vi "Build RPC Request.vi"(10 "Command Params":string[][](array[string]), 11 "VI Name":string) -> (1 "Params":u8, 2 "Unique ID":u16, 3 "Command Buffer":string)   [LabVIEW 2017]
uses:
  <vilib>/Rock Robotics/Network Tables/Make Table Operation.ctl
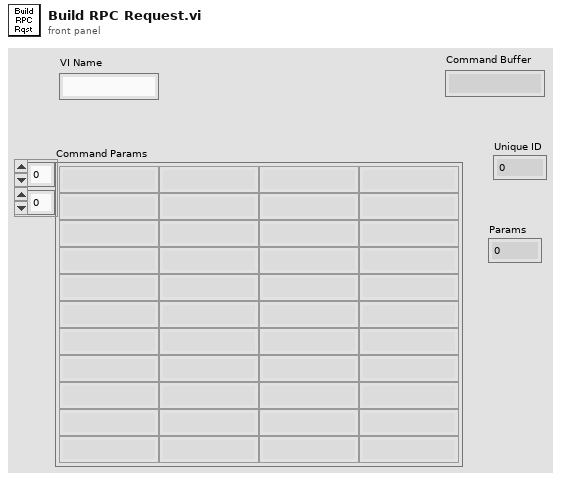
[diagram p1: front panel]
types:
  T1 = typedef "Make Table Operation.ctl" = enum16{"Get or Add Field", "Get Field or Add Temp", "Replace Temp ID", "Get Field ID - No Add", "Get Table Field IDs", "Get Field ID Info", "Move Field to Temp", "Validate", "Remove Field", "Remove All"}
  T2 = typedef "Field ID.ctl" = i32
  T3 = typedef "Field Data.ctl" = cluster{"Dbl":dbl, "String":string, "Type":T4, "Boolean":bool, "Sequence #":T5, "Flags":u8}
  T4 = typedef "Field Type.ctl" = enum8{"Invalid", "Bool", "Numeric", "String", "Raw", "Boolean Array", "Numeric Array", "String Array", "RPC"}
  T5 = typedef "Sequence.ctl" = u16
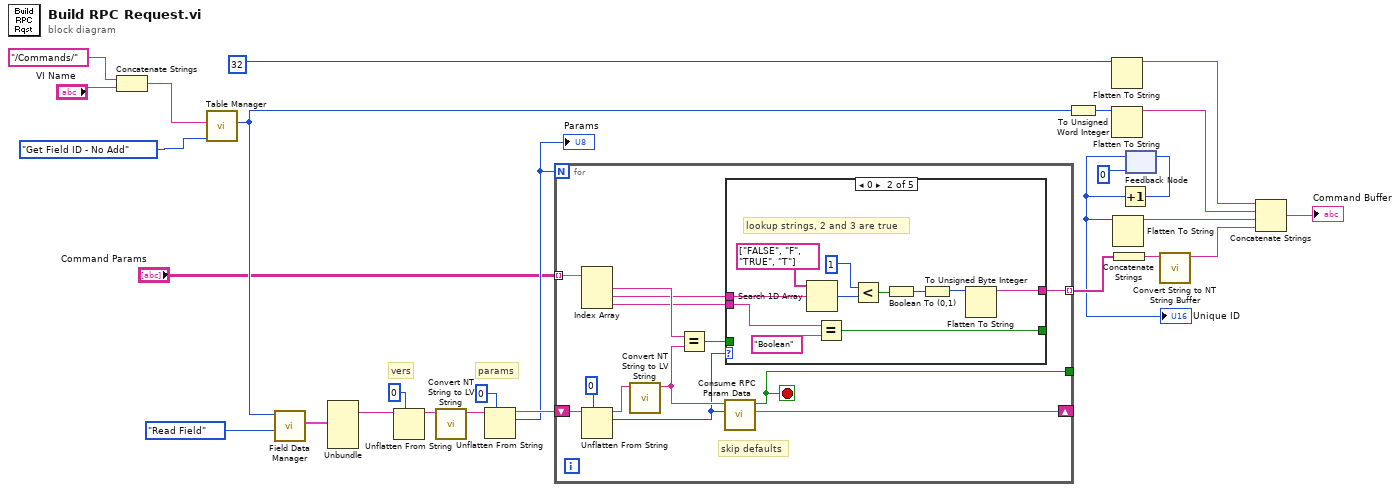
[diagram p0: block diagram]
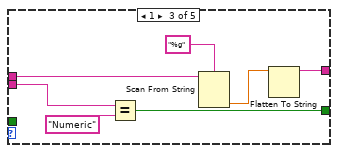
[diagram p3: hidden frame]
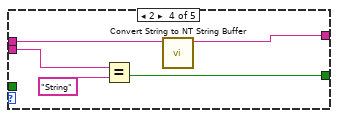
[diagram p4: hidden frame]
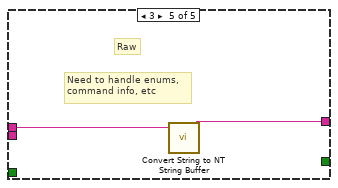
[diagram p5: hidden frame]
diagram:
  # "params"
  # "vers"
  n1 = Concatenate Strings("/Commands/", "VI Name") -> (w2:string)
  n2 = call <vilib>:"Table Manager.vi"("Operation"=Make_Table_Operation."Get Field ID - No Add", "Entry Name"=w2) -> ("Entry ID"=w18:T2)  [unwired: 6 in, 3 out]
  n3 = call <vilib>:"Field Data Manager.vi"("Operation"=enum16{"Update Field", "Read Field"}."Read Field", "Field ID"=w18) -> ("Field Value Out"=w17:T3)  [unwired: 8 in, 1 out]
  n4 = Unbundle(w17) -> ("String"=w12:string)  [unwired: 5 out]
  n5 = Unflatten From String(type=u8 0 ("bytes to read"), binary string=w12) -> (rest of the binary string=w14:string)  [unwired: 3 in, 2 out]
  n6 = call <vilib>:"Convert NT String to LV String.vi"("Buffer in"=w14) -> ("Remaining String"=w16:string)  [unwired: 8 in, 2 out]
  n7 = Unflatten From String(type=u8 0 ("bytes to read"), binary string=w16) -> (rest of the binary string=w11:string, value=w10:u8)  [unwired: 3 in, 1 out]
  "Params" <- w10
  n8 = for {
    N: w10 -> [_]
    shift-right: [w37] -> _
    shift-left: w11 -> [w39]
    tunnel: [w36] -> _
    tunnel: "Command Params" -> [w35] mode=indexing
    tunnel: [w28] -> w6 mode=indexing
    stop <- w36 stop-if-true
    # "skip defaults"
    n9 = Index Array(array=w35) -> (element #1=w33:string, element #2=w30:string, element #3=w29:string)  [unwired: 3 in]
    n10 = Unflatten From String(type=u8 0 ("bytes to read"), binary string=w39) -> (rest of the binary string=w38:string, value=w32:u8)  [unwired: 3 in, 1 out]
    n11 = call <vilib>:"Convert NT String to LV String.vi"("Buffer in"=w38) -> ("Remaining String"=w34:string)  [unwired: 8 in, 2 out]
    n12 = Equal?(x=w33, y=w34) -> (x = y?=w31:bool)
    n13 = call <vilib>:"Consume RPC Param Data.vi"("type"=w32, "RPC String in"=w34) -> ("string out"=w37:string, "Issue"=w36:bool)  [unwired: 6 in, 2 out]
    n14 = case shown="0" w32 {
      tunnel: w31 -> [_ _ _ _ _]
      tunnel: w30 -> [w41 w48 w59 w61 w66]
      tunnel: w29 -> [_ w52 w54 w63 _]
      tunnel: [_ w50 w53 w62 _] -> _
      tunnel: [w41 w42 w56 w60 w65] -> w28
      frame Default {
      }
      frame 0 {
        # "lookup strings, 2 and 3 are true"
        n15 = Search 1D Array(1D array=string[] ["FALSE", "F", "TRUE", "T"], element=w48) -> (index of element=w47:i32)  [unwired: 1 in]
        n16 = Equal?(x=w52, y="Boolean") -> (x = y?=w50:bool)
        n17 = Less?(x=u16 1 ("bytes to read"), y=w47) -> (x < y?=w45:bool)
        n18 = Boolean To (0,1)(Boolean=w45) -> (0, 1=w44:i16)
        n19 = To Unsigned Byte Integer(number=w44) -> (unsigned 8bit integer=w43:u8)
        n20 = Flatten To String(anything=w43) -> (data string=w42:string)  [unwired: 3 in, 2 out]
      }
      frame 1 {
        n21 = Equal?(x=w54, y="Numeric") -> (x = y?=w53:bool)
        n22 = Scan From String(format string="%g", input string=w59) -> (output 1=w57:dbl)  [unwired: 3 in, 3 out]
        n23 = Flatten To String(anything=w57) -> (data string=w56:string)  [unwired: 3 in, 2 out]
      }
      frame 2 {
        n24 = Equal?(x=w63, y="String") -> (x = y?=w62:bool)
        n25 = call <vilib>:"Convert String to NT String Buffer.vi"("LV Buffer"=w61) -> ("NT Buffer"=w60:string)  [unwired: 10 in]
      }
      frame 3 {
        # "Need to handle enums,\ncommand info, etc"
        # "Raw"
        n26 = call <vilib>:"Convert String to NT String Buffer.vi"("LV Buffer"=w66) -> ("NT Buffer"=w65:string)  [unwired: 10 in]
      }
    }
  }
  n27 = To Unsigned Word Integer(number=w18) -> (unsigned 16bit integer=w25:u16)
  n28 = Flatten To String(anything=u8 32 ("bytes to read")) -> (data string=w22:string)  [unwired: 3 in, 2 out]
  n29 = Flatten To String(anything=w25) -> (data string=w21:string)  [unwired: 3 in, 2 out]
  n30 = Concatenate Strings(w6) -> (w7:string)
  n31 = feedback #1(u16 0 ("bytes to read")) -> (w1:u16)
  "Unique ID" <- w1
  n32 = Flatten To String(anything=w1) -> (data string=w20:string)  [unwired: 3 in, 2 out]
  n33 = Increment(x=w1) -> (x+1=w23:u16)
  n34 = feedback-in #1(w23) -> ()
  n35 = call <vilib>:"Convert String to NT String Buffer.vi"("LV Buffer"=w7) -> ("NT Buffer"=w8:string)  [unwired: 10 in]
  n36 = Concatenate Strings(w22, w21, w20, w8) -> (→"Command Buffer":string)
